vi "Sleep State Controlled HVAC System.vi"() -> ()   [LabVIEW 2020]
uses:
  <vilib>/Analysis/baseanly.llb/Mean (DBL).vi
  <vilib>/Analysis/baseanly.llb/Multimode.vi
  <vilib>/Utility/file.llb/Read Delimited Spreadsheet (I64).vi
  <vilib>/measure/mamon.llb/Waveform Peak Detection for 1 Chan.vi
  <vilib>/Analysis/NI_AALBase.lvlib
  <vilib>/measure/NI_MABase.lvlib
  <vilib>/measure/NI_MAPro.lvlib
panel:
  out "HeartRate waveform display unit":waveform(dbl)(graph)
  in  "Input Heart Rate":dbl=10.0 format="%0.2p"
  out "Instantaneous Heartrate Display":i32
  out "Sleep-State Indicator Light":bool
  out "Mean Heart Rate":dbl format="%0.2f"
  out "Resting HeartRate":dbl[](array[numeric]) format="%0.2f"
  in  "ON/OFF Switch":bool
  in  "Temperature Adjuster":dbl
  out "AC Temperature Display":dbl(slide) scale=0.0..30.0
  # "Sleep-State Controlled HVAC System"
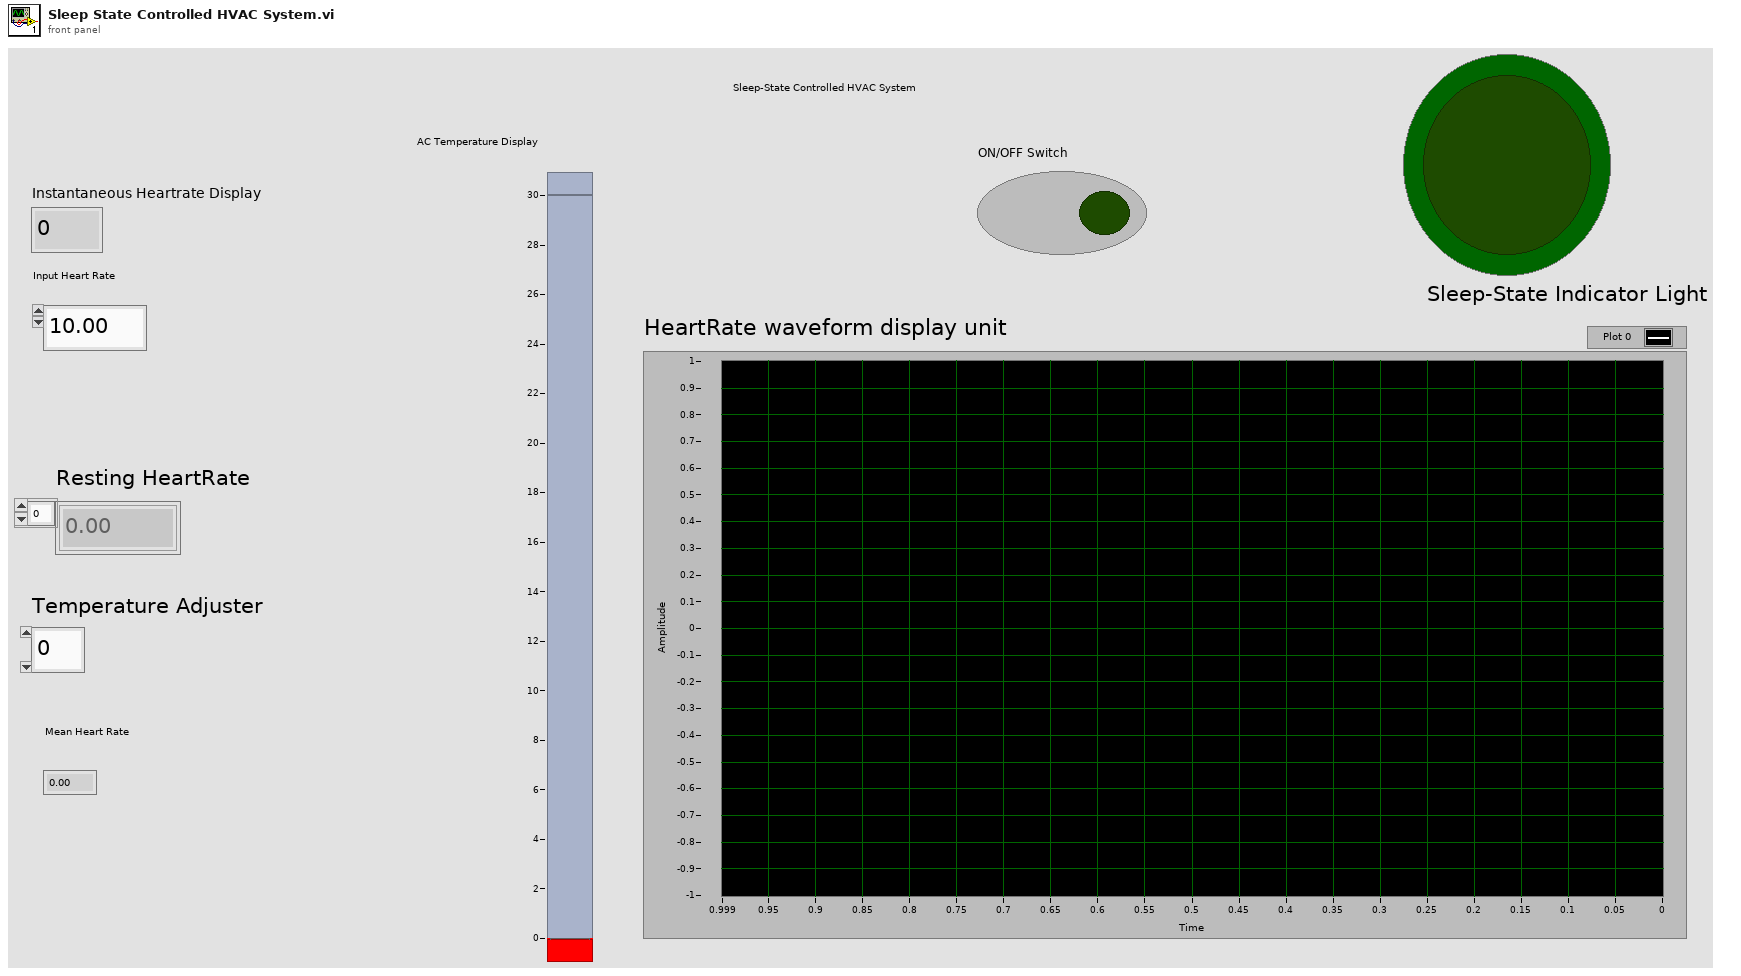
[diagram p1: front panel]
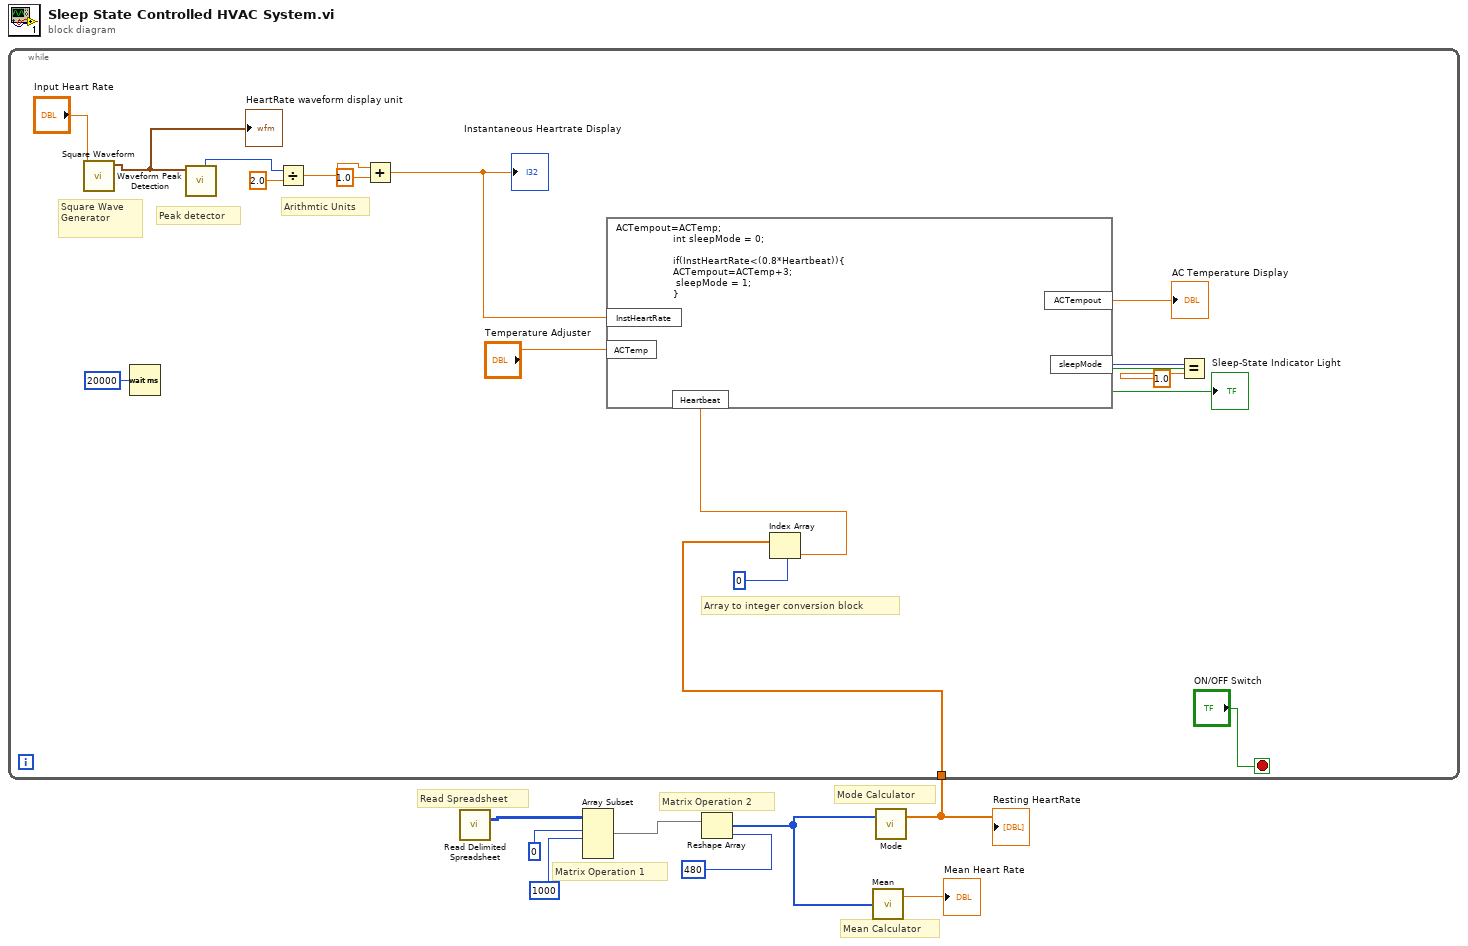
[diagram p0: block diagram]
diagram:
  # "Mean Calculator"
  # "Mode Calculator"
  # "Matrix Operation 2"
  # "Matrix Operation 1"
  # "Read Spreadsheet"
  n1 = call-poly <vilib>:"Read Delimited Spreadsheet.vi"() -> ("all rows"=w6:i64[][])  [unwired: 10 in, 5 out]
  n2 = Array Subset(array=w6, index (row)=0 ("index"), length (row)=1000 ("length")) -> (w5:i64[][])  [unwired: 2 in]
  n3 = Reshape Array(w5, 480 ("dimension size")) -> (w3:i64[])
  n4 = call-poly <vilib>:"Mean.vi"("X"=w3) -> ("mean"=→"Mean Heart Rate":dbl)  [unwired: 1 out]
  n5 = call-poly <vilib>:"Mode.vi"("X"=w3) -> ("Modes"=w1:dbl[])  [unwired: 1 in, 1 out]
  "Resting HeartRate" <- w1
  n6 = while {
    tunnel: w1 -> [w20]
    stop <- "ON/OFF Switch" stop-if-true
    # "Array to integer conversion block"
    # "Arithmtic Units"
    # "Peak detector"
    # "Square Wave Generator"
    n7 = call <vilib>:"Square Waveform.vi"("frequency"="Input Heart Rate") -> ("signal out"=w15:waveform(dbl))  [unwired: 9 in, 1 out]
    "HeartRate waveform display unit" <- w15
    n8 = Wait (ms)(milliseconds to wait=u32 20000) -> ()  [unwired: 1 out]
    n9 = call-poly <vilib>:"Waveform Peak Detection.vi"("Signal In"=w15) -> ("# found"=w13:i32)  [unwired: 6 in, 4 out]
    n10 = Divide(x=w13, y=2.0) -> (x/y=w11:dbl)
    n11 = Add(x=w11, y=1.0) -> (x+y=w9:dbl)
    "Instantaneous Heartrate Display" <- w9
    n12 = Index Array(array=w20, index=0) -> (element=w21:dbl)
    n13 = formula code="ACTempout=ACTemp;\n                   int sleepMode = 0;\n\n                   if(InstHeartRate<(0.8*Heartbeat)){\n                   ACTempout=ACTemp+3;\n                    sleepMode = 1;\n                   }"("InstHeartRate"=w9, "ACTemp"="Temperature Adjuster", "Heartbeat"=w21) -> ("ACTempout"=→"AC Temperature Display":dbl, "sleepMode"=w17:i32)
    n14 = Equal?(x=w17, y=1.0) -> (x = y?=→"Sleep-State Indicator Light":bool)
  }
